vi "getMeasSetforTemperature.vi"(0 "measSetId":string="5930", 1 "Database":T1={"DB name"="zaop", "UID"="sel00752", "password"="rhkdwo7978"}, 2 "Log file":path=path "C:/Temp/Log/test.txt", 3 "error in (no error)":errorcluster) -> (7 "meas_setting array":T2[](array[typedef])=[{"measSetId"=5930, "measSetComments"="Beamstyle", "probeId"=13441.0, "beamstyleIndex"=5, "txFrequencyHz"=3636400.0, "focusRangeCm"=4.5, "maxTxVoltageVolt"=100.0, "ceilTxVoltageVolt"=100.0, "profTxVoltageVolt"=62.0, "totalVoltagePt"=20, "numMeasVoltage"=12, "numTxElements"=34, "txpgWaveformStyle"=2, "numTxCycles"=4.0, "elevAperIndex"=0, "zStartDistCm"=1.9, "zMeasNum"=65, "IsTxAperModulationEn"=0, "DTxFreqIndex"=0, "VTxIndex"=0, "IsCPAEn"=0, "SysPulserSelA"=0, "TxPulseRleA"=""}] {"zStartDistCm" format="%.2f"; "numTxCycles" format="%.1f"; "profTxVoltageVolt" format="%#_1g"; "ceilTxVoltageVolt" format="%.2f"; "maxTxVoltageVolt" format="%.2f"; "focusRangeCm" format="%.1f"; "txFrequencyHz" format="%.2f"}, 9 "error out":errorcluster)   [LabVIEW 2016]
doc: "Retrieves an array of measurement settings and a cluster of accessory parameters from the database. The input measSetId list may include multiple IDs separated by commas, and ranges specified with dashes. One cluster of data is retrieved from meas_setting for each ID in the list, and an array of these clusters is returned. The input measIntenParamId is used to retrieve data from table meas_inten_param. Errors are reported if the retrieved measSetIds or measIntenParamId don't match the input values."
uses:
  type def/measSetting.ctl
  type def/Database.ctl
  TemperatureMeasure/Thermal_type.vi
panel:
  out "배열":i32[](array[numeric])
  out "연결된 문자열":string
  out "meaSetId(Volt)":i32[](array[numeric])
  out "meaSetId(SA)":i32[](array[numeric])
  in  "floating-point type conversion":string[][](table)=[["extended", "5", "12"], ["double", "5", "9"], ["single", "5", "5"]]
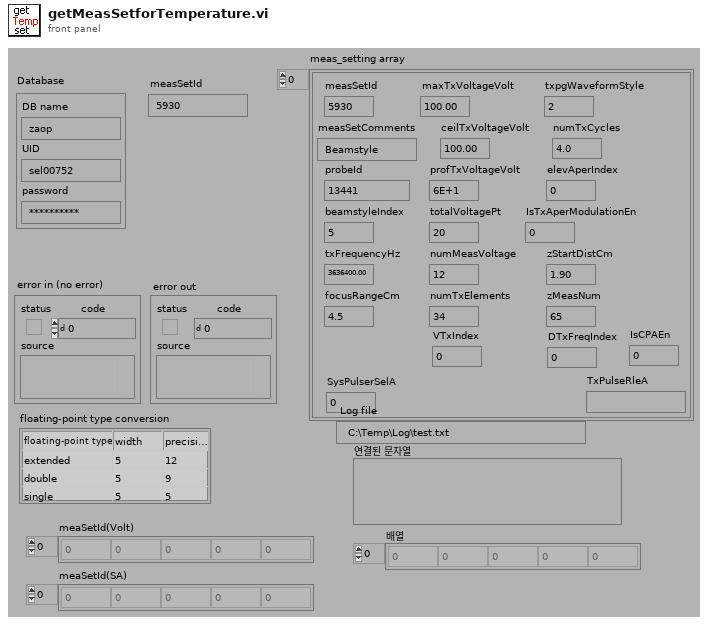
[diagram p1: front panel]
types:
  T1 = typedef "Database.ctl" = cluster{"DB name":string, "UID":string, "password":string}
  T2 = typedef "measSetting.ctl" = cluster{"measSetId":i32, "measSetComments":string, "probeId":sgl, "beamstyleIndex":i16, "txFrequencyHz":sgl, "focusRangeCm":sgl, "maxTxVoltageVolt":sgl, "ceilTxVoltageVolt":sgl, "profTxVoltageVolt":dbl, "totalVoltagePt":i8, "numMeasVoltage":i8, "numTxElements":i16, "txpgWaveformStyle":i8, "numTxCycles":sgl, "elevAperIndex":i8, "zStartDistCm":sgl, "zMeasNum":i8, "IsTxAperModulationEn":i8, "DTxFreqIndex":i16, "VTxIndex":i8, "IsCPAEn":i16, "SysPulserSelA":i16, "TxPulseRleA":string}
  T3 = cluster{"status":bool, "code":i32, "text":string}
  T4 = typedef "Connection - Recordset reference.ctl" = cluster{"Connection":refnum<k7>, "Recordset":refnum<k7>}
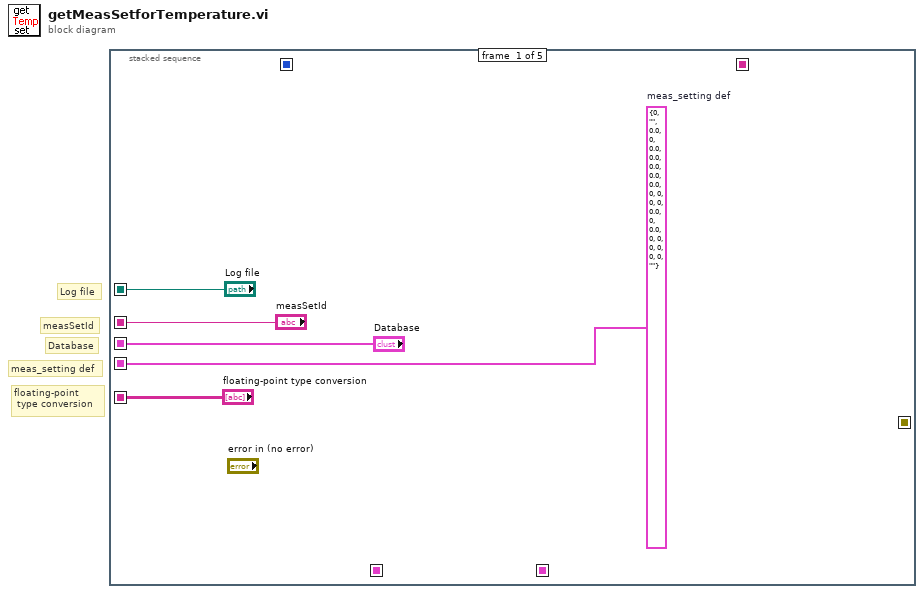
[diagram p0: block diagram]
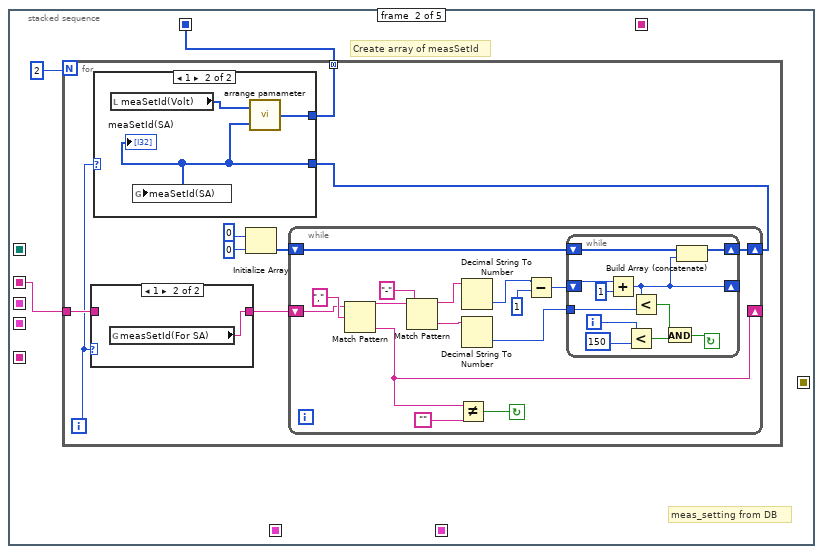
[diagram p2: hidden frame]
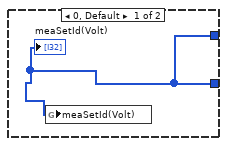
[diagram p3: hidden frame]
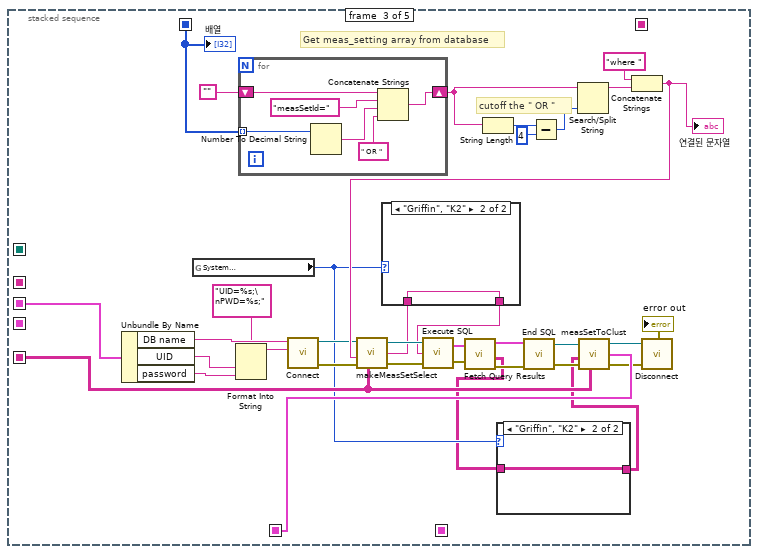
[diagram p5: hidden frame]
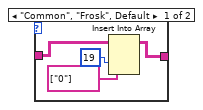
[diagram p6: hidden frame]
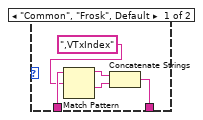
[diagram p7: hidden frame]
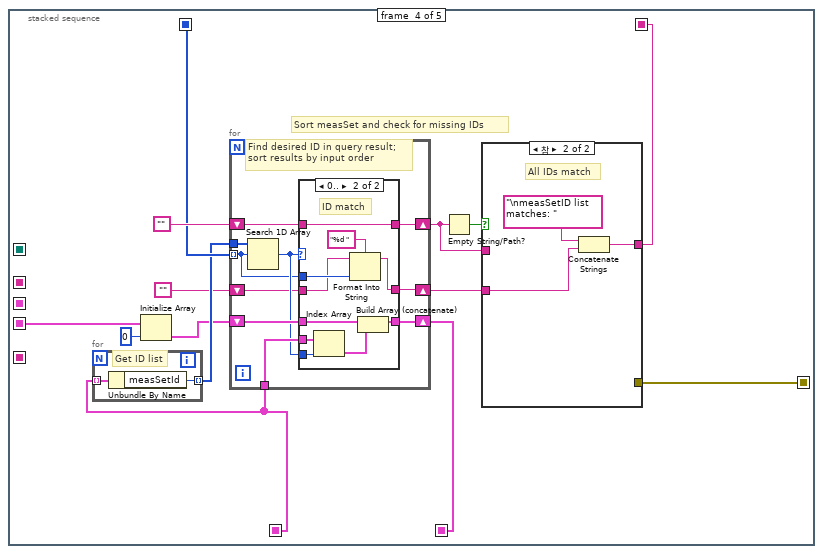
[diagram p8: hidden frame]
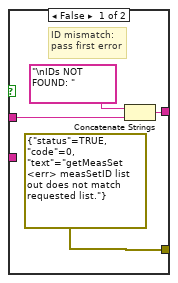
[diagram p9: hidden frame]
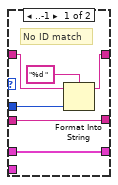
[diagram p10: hidden frame]
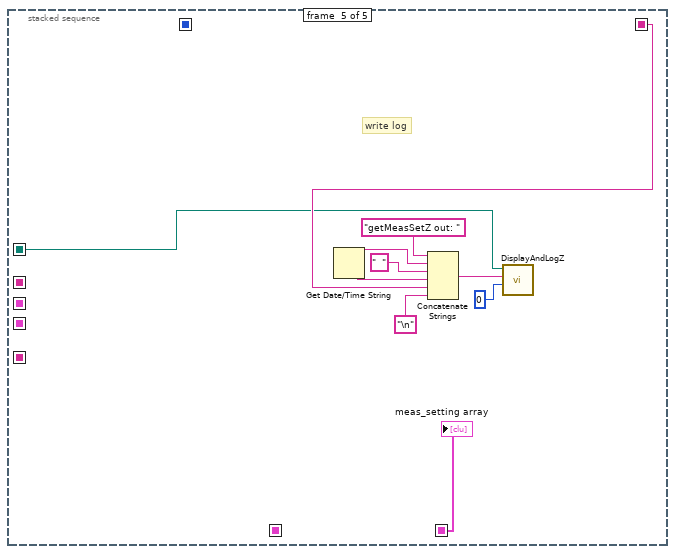
[diagram p11: hidden frame]
diagram:
  # "meas_setting def"
  # "floating-point\n type conversion"
  # "Database"
  # "Log file"
  # "measSetId"
  n1 = stacked-sequence {
    seq-local: [_ w6 _ _ _] -> [_ _ w54 w110 _]
    seq-local: [w1 _ _ _ _] -> [_ _ _ w101 _]
    seq-local: ["measSetId" _ _ _ _] -> [_ w8 _ _ _]
    seq-local: ["Database" _ _ _ _] -> [_ _ w60 _ _]
    seq-local: [_ _ w58 _ _] -> [_ _ _ w108 _]
    seq-local: [_ _ _ w112 _] -> [_ _ _ _ w153]
    seq-local: ["Log file" _ _ _ _] -> [_ _ _ _ w152]
    seq-local: [_ _ _ w103 _] -> [_ _ _ _ w151]
    seq-local: ["floating-point type conversion" _ _ _ _] -> [_ _ w59 _ _]
    seq-local: [_ _ _ w102 _] -> [_ _ _ _ _]
    frame #0 {
      w1 = T2 {"measSetId"=0, "measSetComments"="", "probeId"=0.0, "beamstyleIndex"=0, "txFrequencyHz"=0.0, "focusRangeCm"=0.0, "maxTxVoltageVolt"=0.0, "ceilTxVoltageVolt"=0.0, "profTxVoltageVolt"=0.0, "totalVoltagePt"=0, "numMeasVoltage"=0, "numTxElements"=0, "txpgWaveformStyle"=0, "numTxCycles"=0.0, "elevAperIndex"=0, "zStartDistCm"=0.0, "zMeasNum"=0, "IsTxAperModulationEn"=0, "DTxFreqIndex"=0, "VTxIndex"=0, "IsCPAEn"=0, "SysPulserSelA"=0, "TxPulseRleA"=""}  # meas_setting def
    }
    frame #1 {
      # "meas_setting from DB"
      # "Create array of measSetId"
      n2 = for {
        N: 2 -> [_]
        tunnel: w8 -> [w13]
        tunnel: [w9] -> w6 mode=concatenating
        i -> [w11]
        n3 = case shown="1" w11 {
          tunnel: [w21 w22] -> w12
          tunnel: w13 -> [w21 _]
          frame 0, Default {
          }
          frame 1 {
            n4 = global read "Thermal_type.vi" "measSetId(For SA)"() -> (w22:string)
          }
        }
        n5 = Initialize Array(0, 0) -> (w14:i32[])
        n6 = while {
          shift-left: w14 -> [w24]
          shift-right: [w23] -> w10
          shift-left: w12 -> [w33]
          shift-right: [w30] -> _
          stop <- w34 continue-if-true
          n7 = Match Pattern(string=w33, regular expression=",") -> (before substring=w31:string, after substring=w30:string)  [unwired: 1 in, 2 out]
          n8 = Match Pattern(string=w31, regular expression="-") -> (before substring=w35:string, after substring=w29:string)  [unwired: 1 in, 2 out]
          n9 = Not Equal?(x=w30, y="") -> (x != y?=w34:bool)
          n10 = Decimal String To Number(string=w35) -> (number=w27:i32)  [unwired: 2 in, 1 out]
          n11 = Decimal String To Number(string=w29) -> (number=w25:i32)  [unwired: 2 in, 1 out]
          n12 = Subtract(x=w27, y=1) -> (x-y=w26:i32)
          n13 = while {
            shift-left: w24 -> [w40]
            shift-right: [w39] -> w23
            tunnel: w25 -> [w41]
            shift-left: w26 -> [w44]
            shift-right: [w38] -> _
            i -> [w43]
            stop <- w42 continue-if-true
            n14 = Add(x=w44, y=1) -> (x+y=w38:i32)
            n15 = Less?(x=w43, y=150) -> (x < y?=w46:bool)
            n16 = Less?(x=w38, y=w41) -> (x < y?=w45:bool)
            n17 = And(x=w45, y=w46) -> (x .and. y?=w42:bool)
            n18 = Build Array (concatenate)(w40, w38) -> (w39:i32[])
          }
        }
        n19 = case shown="1" w11 {
          tunnel: w10 -> [w17 w19]
          tunnel: [w17 w18] -> w9
          frame 0, Default {
            n20 = global write "Thermal_type.vi" "meaSetId(Volt)"(w17) -> ()
            "meaSetId(Volt)" <- w17
          }
          frame 1 {
            n21 = local read "meaSetId(Volt)"() -> (w20:i32[])
            n22 = global write "Thermal_type.vi" "meaSetId(SA)"(w19) -> ()
            n23 = call "arrange pamameter.vi"("meaSetId(SA)"=w19, "meaSetId(Volt)"=w20) -> ("Arrange MeasSetid"=w18:i32[])
            "meaSetId(SA)" <- w19
          }
        }
      }
    }
    frame #2 {
      # "cutoff the \" OR \""
      # "Get meas_setting array from database"
      n24 = Unbundle By Name(w60) -> ("DB name"=w83:string, "UID"=w75:string, "password"=w74:string)
      n25 = global read "Thermal_type.vi" "System \nSelection"() -> (w51:enum32{"Common", "Frosk", "Griffin", "K2"})
      n26 = Format Into String(format string="UID=%s;\nPWD=%s;" ("Format String"), w75, w74) -> (resulting string=w82:string)  [unwired: 2 in, 1 out]
      n27 = for {
        tunnel: w54 -> [w95] mode=indexing
        shift-right: [w96] -> w66
        shift-left: "" -> [w100]
        n28 = Number To Decimal String(number=w95) -> (decimal integer string=w98:string)  [unwired: 1 in]
        n29 = Concatenate Strings(w100, "measSetId=", w98, " OR ") -> (w96:string)
      }
      n30 = call <vilib>:"Connect.vi"("connection parameters"=w82, "data source name"=w83) -> ("error out"=w79:errorcluster, "Connection"=w78:refnum<k7>)  [unwired: 2 in]
      n31 = String Length(string=w66) -> (length=w77:i32)
      n32 = Subtract(x=w77, y=4) -> (x-y=w64:i32)
      n33 = Search/Split String(string=w66, offset (0)=w64) -> (substring before match=w63:string)  [unwired: 1 in, 2 out]
      n34 = Concatenate Strings("where ", w63) -> (w80:string)
      "연결된 문자열" <- w80
      n35 = call "makeMeasSetSelect.vi"("connection reference"=w78, "condition"=w80, "floating-point type conversion"=w59, "error in"=w79) -> ("connection reference"=w73:refnum<k7>, "select sql statement"=w53:string, "error out"=w72:T3)  [unwired: 2 in]
      n36 = case shown="\"Griffin\", \"K2\"" w51 {
        tunnel: w53 -> [w93 w94]
        tunnel: [w89 w94] -> w52
        frame "Common", "Frosk", Default {
          n37 = Match Pattern(string=w93, regular expression=",VTxIndex") -> (before substring=w91:string, after substring=w90:string)  [unwired: 1 in, 2 out]
          n38 = Concatenate Strings(w91, w90) -> (w89:string)
        }
        frame "Griffin", "K2" {
        }
      }
      n39 = call <vilib>:"Execute SQL.vi"("error in (no error)"=w72, "SQL Statement"=w52, "Connection"=w73) -> ("error out"=w61:errorcluster, "reference"=w71:T4)
      n40 = call <vilib>:"Fetch Query Results.vi"("reference"=w71, "error in (no error)"=w61) -> ("reference"=w70:T4, "query"=w50:string[][], "error out"=w69:errorcluster)  [unwired: 1 out]
      n41 = case shown="\"Griffin\", \"K2\"" w51 {
        tunnel: w50 -> [w85 w88]
        tunnel: [w84 w88] -> w49
        frame "Common", "Frosk", Default {
          n42 = Insert Into Array(array=w85, index (col)=19 ("인덱스 (행)"), new element=string[] ["0"] ("새 원소/부분배열")) -> (w84:string[][])  [unwired: 1 in]
        }
        frame "Griffin", "K2" {
        }
      }
      n43 = call <vilib>:"End SQL.vi"("error in (no error)"=w69, "reference"=w70) -> ("error out"=w68:errorcluster, "Connection"=w67:refnum<k7>)
      n44 = call "measSetToClust.vi"("connection reference"=w67, "query results"=w49, "floating-point type conversion"=w59, "error in"=w68) -> ("connection reference"=w57:refnum<k7>, "meas_setting array"=w58:T2[], "error out"=w56:T3)  [unwired: 2 in]
      n45 = call <vilib>:"Disconnect.vi"("error in (no error)"=w56, "connection"=w57) -> ("error out"=→"error out":errorcluster)  [unwired: 1 in]
      "배열" <- w54
    }
    frame #3 {
      # "Sort measSet and check for missing IDs"
      n46 = for {
        tunnel: w108 -> [w116] mode=indexing
        tunnel: [w115] -> w109 mode=indexing
        # "Get ID list"
        n47 = Unbundle By Name(w116) -> ("measSetId"=w115:i32)
      }
      n48 = Initialize Array(w101, 0 ("Dimension Size")) -> (w106:T2[])
      n49 = for {
        tunnel: w110 -> [w128] mode=indexing
        shift-right: [w124] -> w111
        shift-left: "" -> [w125]
        tunnel: w109 -> [w133]
        tunnel: w108 -> [w130]
        shift-right: [w131] -> w103
        shift-left: w106 -> [w132]
        shift-right: [w126] -> w104
        shift-left: "" -> [w127]
        # "Find desired ID in query result;\nsort results by input order"
        n50 = Search 1D Array(1D array=w133, element=w128) -> (index of element=w129:i32)  [unwired: 1 in]
        n51 = case shown="0.." w129 {
          tunnel: w132 -> [w139 w149]
          tunnel: [w139 w148] -> w131
          tunnel: w130 -> [_ w147]
          tunnel: w129 -> [_ w146]
          tunnel: w128 -> [w135 w142]
          tunnel: w127 -> [w138 w141]
          tunnel: [w138 w140] -> w126
          tunnel: w125 -> [w136 w144]
          tunnel: [w134 w144] -> w124
          frame ..-1 {
            # "No ID match"
            n52 = Format Into String(format string="%d " ("Format String"), initial string=w136, w135) -> (resulting string=w134:string)  [unwired: 1 in, 1 out]
          }
          frame 0.. {
            # "ID match"
            n53 = Index Array(array=w147, index=w146) -> (element=w145:T2)
            n54 = Format Into String(format string="%d " ("Format String"), initial string=w141, w142) -> (resulting string=w140:string)  [unwired: 1 in, 1 out]
            n55 = Build Array (concatenate)(w149, w145) -> (w148:T2[])
          }
        }
      }
      n56 = Empty String/Path?(string/path=w111) -> (empty?=w113:bool)
      n57 = case shown="참" w113 {
        tunnel: [w118 w122] -> w112
        tunnel: w111 -> [w119 _]
        tunnel: [T3 {"status"=TRUE, "code"=0, "text"="getMeasSet <err> measSetID list out does not match requested list."} ("error out") _] -> w102
        tunnel: w104 -> [_ w121]
        frame False {
          # "ID mismatch:\npass first error"
          n58 = Concatenate Strings("\nIDs NOT FOUND: " ("Substring"), w119) -> (w118:string)
        }
        frame True {
          # "All IDs match"
          n59 = Concatenate Strings("\nmeasSetID list matches: " ("Substring"), w121) -> (w122:string)
        }
      }
    }
    frame #4 {
      # "write log"
      n60 = Get Date/Time String() -> (date string=w158:string, time string=w156:string)  [unwired: 3 in]
      n61 = Concatenate Strings("getMeasSetZ out: " ("Substring"), w158, "  ", w156, w153, "\n" ("Substring")) -> (w154:string)
      n62 = call "DisplayAndLogZ.vi"("Log file"=w152, "message"=w154, "action (0: log+display)"=u16 0) -> ()  [unwired: 5 in, 1 out]
      "meas_setting array" <- w151
    }
  }
